vi "ADC Number.vi"(4 "AnalogIn in":refnum<class "AI.lvclass">) -> (7 "ADC #":T1=-1)   [LabVIEW 2020, in "CTI.lvlib" / "AI.lvclass"]
uses:
  AI.lvclass
  AI.lvclass/AI.ctl
  ADC Number.ctl
  CTI.lvlib
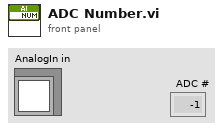
[diagram p1: front panel]
types:
  T1 = typedef "CTI.lvlib/ADC Number.ctl" = i8
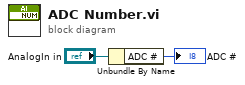
[diagram p0: block diagram]
diagram:
  n1 = Unbundle By Name("AnalogIn in") -> ("ADC #"=→"ADC #":T1)
